vi "Dashboard Main (BEDPC-GB8-7's conflicted copy 2019-03-26).vi"() -> ()   [LabVIEW 2018]
uses:
  <vilib>/Utility/miscctls.llb/LVRowAndColumnTypeDef.ctl
  <vilib>/event_ctls.llb/eventvkey.ctl
  <vilib>/Rock Robotics/Network Tables/NT Read Boolean.vi
  <vilib>/Rock Robotics/Network Tables/NT Write Boolean.vi
  <vilib>/Rock Robotics/Network Tables/NT Read Numeric Array.vi
  <vilib>/Rock Robotics/WPI/Dashboard/WPI_DashboardLogging Global.vi
panel:
  in  "Camera Settings Right":T1={"Frame Rate"=30, "Compression"=30, "Size"=1, "DB Camera Config"=FALSE} {"Frame Rate" scale=1.0..30.0; "Compression" scale=100.0..-1.0; "Size" items=["640x480", "320x240", "160x120"]}
  in  "Camera Name Right":string(combo)="No Camera Selection"
  out "Camera Perf":string
  in  "Camera Settings":T1={"Frame Rate"=30, "Compression"=30, "Size"=1, "DB Camera Config"=FALSE} {"Frame Rate" scale=1.0..30.0; "Compression" scale=100.0..-1.0; "Size" items=["640x480", "320x240", "160x120"]}
  in  "TCP":refnum<k5>
  in  "Rec Mode":enum32{"Stop", "Record", "Playback"}(radio)
  out "Image Message":string="Timeout in Camera Communications"
  in  "Dashboard Tab":T2(tab)
  out "Limelight Target State":bool
  out "Hatch Open":bool
  out "Hatch Extend":bool
  out "Cargo Piston":bool
  in  "Zero Yaw":bool
  out "Yaw":dbl
  out "Cont Yaw":dbl
  out "LowerLimit":bool
  out "UpperLimit":bool
  out "HAB Retracting limit":bool
  out "HAB Extending limit":bool
  in  "Select Auto":string(combo)="Select Autonomous ..."
  out "NT Connection":bool
  out "Mode":T3(ring)=enum."Auto Disabled"
  out "Right Camera Perf":cluster{"Bandwidth (Mbps)":dbl, "FPS":dbl}
  out "Lift Auto Position":u16(ring) items=["Cargo 1", "Hatch 1", "Cargo 2", "Hatch 2", "Cargo 3", "Hatch 3"]
  out "Wheel Rates":T4
  out "Wheel Angles":T4
  out "Y-Velocity":dbl
  out "X-Velocity":dbl
  out "Wheel Positions":T4
  out "Tree":string(tree)
  in  "Test Slider":dbl(slide) scale=0.0..100.0 scale format="%#_3g"
  in  "On/Off":bool caption="Solenoid"
  in  "Test Name":u16(ring) items=["Select the test to run..."]
  in  "Test Tree":string(tree)
  in  "Motor":cluster{"Value":dbl, "Enable":bool} {"Value" scale=-1.0..1.0 scale format="%#_3g"}
  out "Progress":T5 {"Test Progress" scale=0.0..100.0}
  in  "Rev/Fwd":cluster{"Forward":bool, "Reverse":bool}
  in  "Test Ring":u16(ring) items=["Monochrome", "Color"]
  in  "CheckList":i32(listbox)
  out "Cmd Status":string
  in  "Execute Command":bool
  in  "Command Params":string[][](table)
  in  "Command Selection":i32(listbox)
  out "Camera Image":T6(plugin-control)
  in  "Camera Name":string(combo)="No Camera Selection"
  # "HW"
  # "HW"
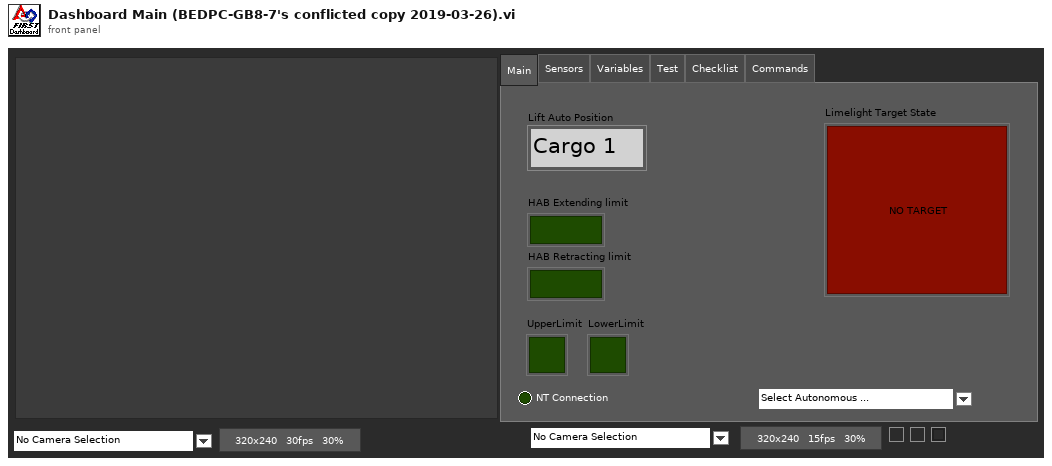
[diagram p1: front panel]
types:
  T1 = cluster{"Frame Rate":i32, "Compression":i32, "Size":u16, "DB Camera Config":bool}
  T2 = enum32{"Main", "Sensors", "Variables", "Test", "Checklist", "Commands"}
  T3 = enum8{"Tele-Op Disabled", "Tele-Op Enabled", "Auto Disabled", "Auto Enabled", "Test Disabled", "Test Enabled", "Disconnected", "No Code", "E-Stop"}
  T4 = cluster{"FrontLeft":dbl, "FrontRight":dbl, "BackLeft":dbl, "BackRight":dbl}
  T5 = cluster{"Test Progress":u8, "Test Progress Text":string}
  T6 = typedef "IMAQ Image.ctl" = refnum<image>
  T7 = cluster{"Save Path":path, "Interval (s)":dbl, "Keep":i32}
  T8 = enum32{"Drive", "Camera", "Basic", "Custom", "Test", "Commands", "Checklist", "Variables"}
  T9 = typedef "Image Type" = u32
  T10 = cluster{"IDs":cluster{"RPC field ID":u16, "Unique ID":u16}, "String":string}
  T11 = cluster{"Error Strings":string, "Disable Counts":cluster{u16, u16}, "Rail Faults":cluster{u16, u16, u16}, "Robot IP":string, "DB Mode":u8, "Event Info":cluster{"Name":string, "Type":u8, "Number":u16, "Replay":u8}}
  T12 = cluster{"Storage":cluster{"Disk Free":u64, "RAM Block":u32, "RAM free":u32}, "CPU Utilization":cluster{"CPU % ISR":sgl, "CPU % Time Crit":sgl, "CPU % Timed Str":sgl, "CPU % High":sgl, "CPU % Above":sgl, "CPU % Normal":sgl, "CPU % Low":sgl}, "CAN":cluster{"% Bus Utilization":sgl, "Bus Off Cnt":u32, "TX_FIFO Full Cnt":u32, "Receive Error Cnt":u8, "Transmit Error Cnt":u8}, "HID":cluster{"HID Outputs":u32, "Rumble Low":u16, "Rumble High":u16}[]}
  T13 = cluster{"Status bits":cluster{"Test Mode":bool, "Autonomous":bool, "Enabled":bool, "Code Start":bool, "Brownout":bool, "Reserved 2":bool, "Reserved 3":bool, "E-Stop":bool}, "Code Trace":cluster{"Disabled":bool, "TeleOp":bool, "Auto":bool, "Test":bool}, "Controller Type":enum16{"unknown", "cRIO", "roboRio"}, "Code?":enum16{"unknown", "noCode", "code"}, "Battery V":dbl}
  T14 = cluster{"Control Bits":cluster{"TestMode":bool, "Autonomous":bool, "Enabled":bool, "FMS Present":bool, bool, bool, bool, "E-Stop":bool}, "Team Station ":u8, "Countdown":sgl, "Joystick Values":cluster{"Axes":dbl[], "Buttons":bool[], "POVs":i16[]}[]}
  T15 = cluster{"Numeric":dbl, "Numeric":dbl, "Numeric":dbl, "Numeric":dbl}
  T16 = cluster{"Global Rectangle":i32[], "Contours":cluster{"Contour Type":u32, "ROI Type":u32, "Points":i32[]}[]}
  T17 = cluster{"Camera Name":string, string, "Saved DB Images Info":cluster{"Save Path":path, "Interval (s)":dbl, "Keep":i32}}
  T18 = cluster{"Camera Name Right":string, string, "Saved DB Images Info":cluster{"Save Path":path, "Interval (s)":dbl, "Keep":i32}}
  T19 = cluster{"Operation":enum16{"Update", "Clear"}, "Color Box":u32}[]
  T20 = typedef "eventvkey.ctl" = enum16{"ASCII", "Enter", "Return", "Shift", "Ctrl", "Alt", "Cmd", "Opt", "Caps", "NumLock", "Clear", "Break", "Up", "Down", "Left", "Right", "Insert", "Delete", "Home", "End", "PageUp", "PageDown", "Escape", "Help", "Pause", "ScrollLock", "F1", "F2", "F3", "F4", "F5", "F6", "F7", "F8", "F9", "F10", "F11", "F12", "F13", "F14", "F15", "F16", "F17", "F18", "F19", "F20", "F21", "F22", "F23", "F24", "Play", "VolumeUp", "VolumeDown", "Mute", "Two Byte Char"}
  T21 = cluster{"Operation":enum16{"Update", "Clear"}, "Color Box":u32}
  T22 = typedef "LVRowAndColumnTypeDef.ctl" = cluster{"Row":i32, "Column":i32}
  T23 = cluster{"Shift":bool, "Ctrl":bool, "Alt":bool, "Cmd":bool, "Opt":bool}
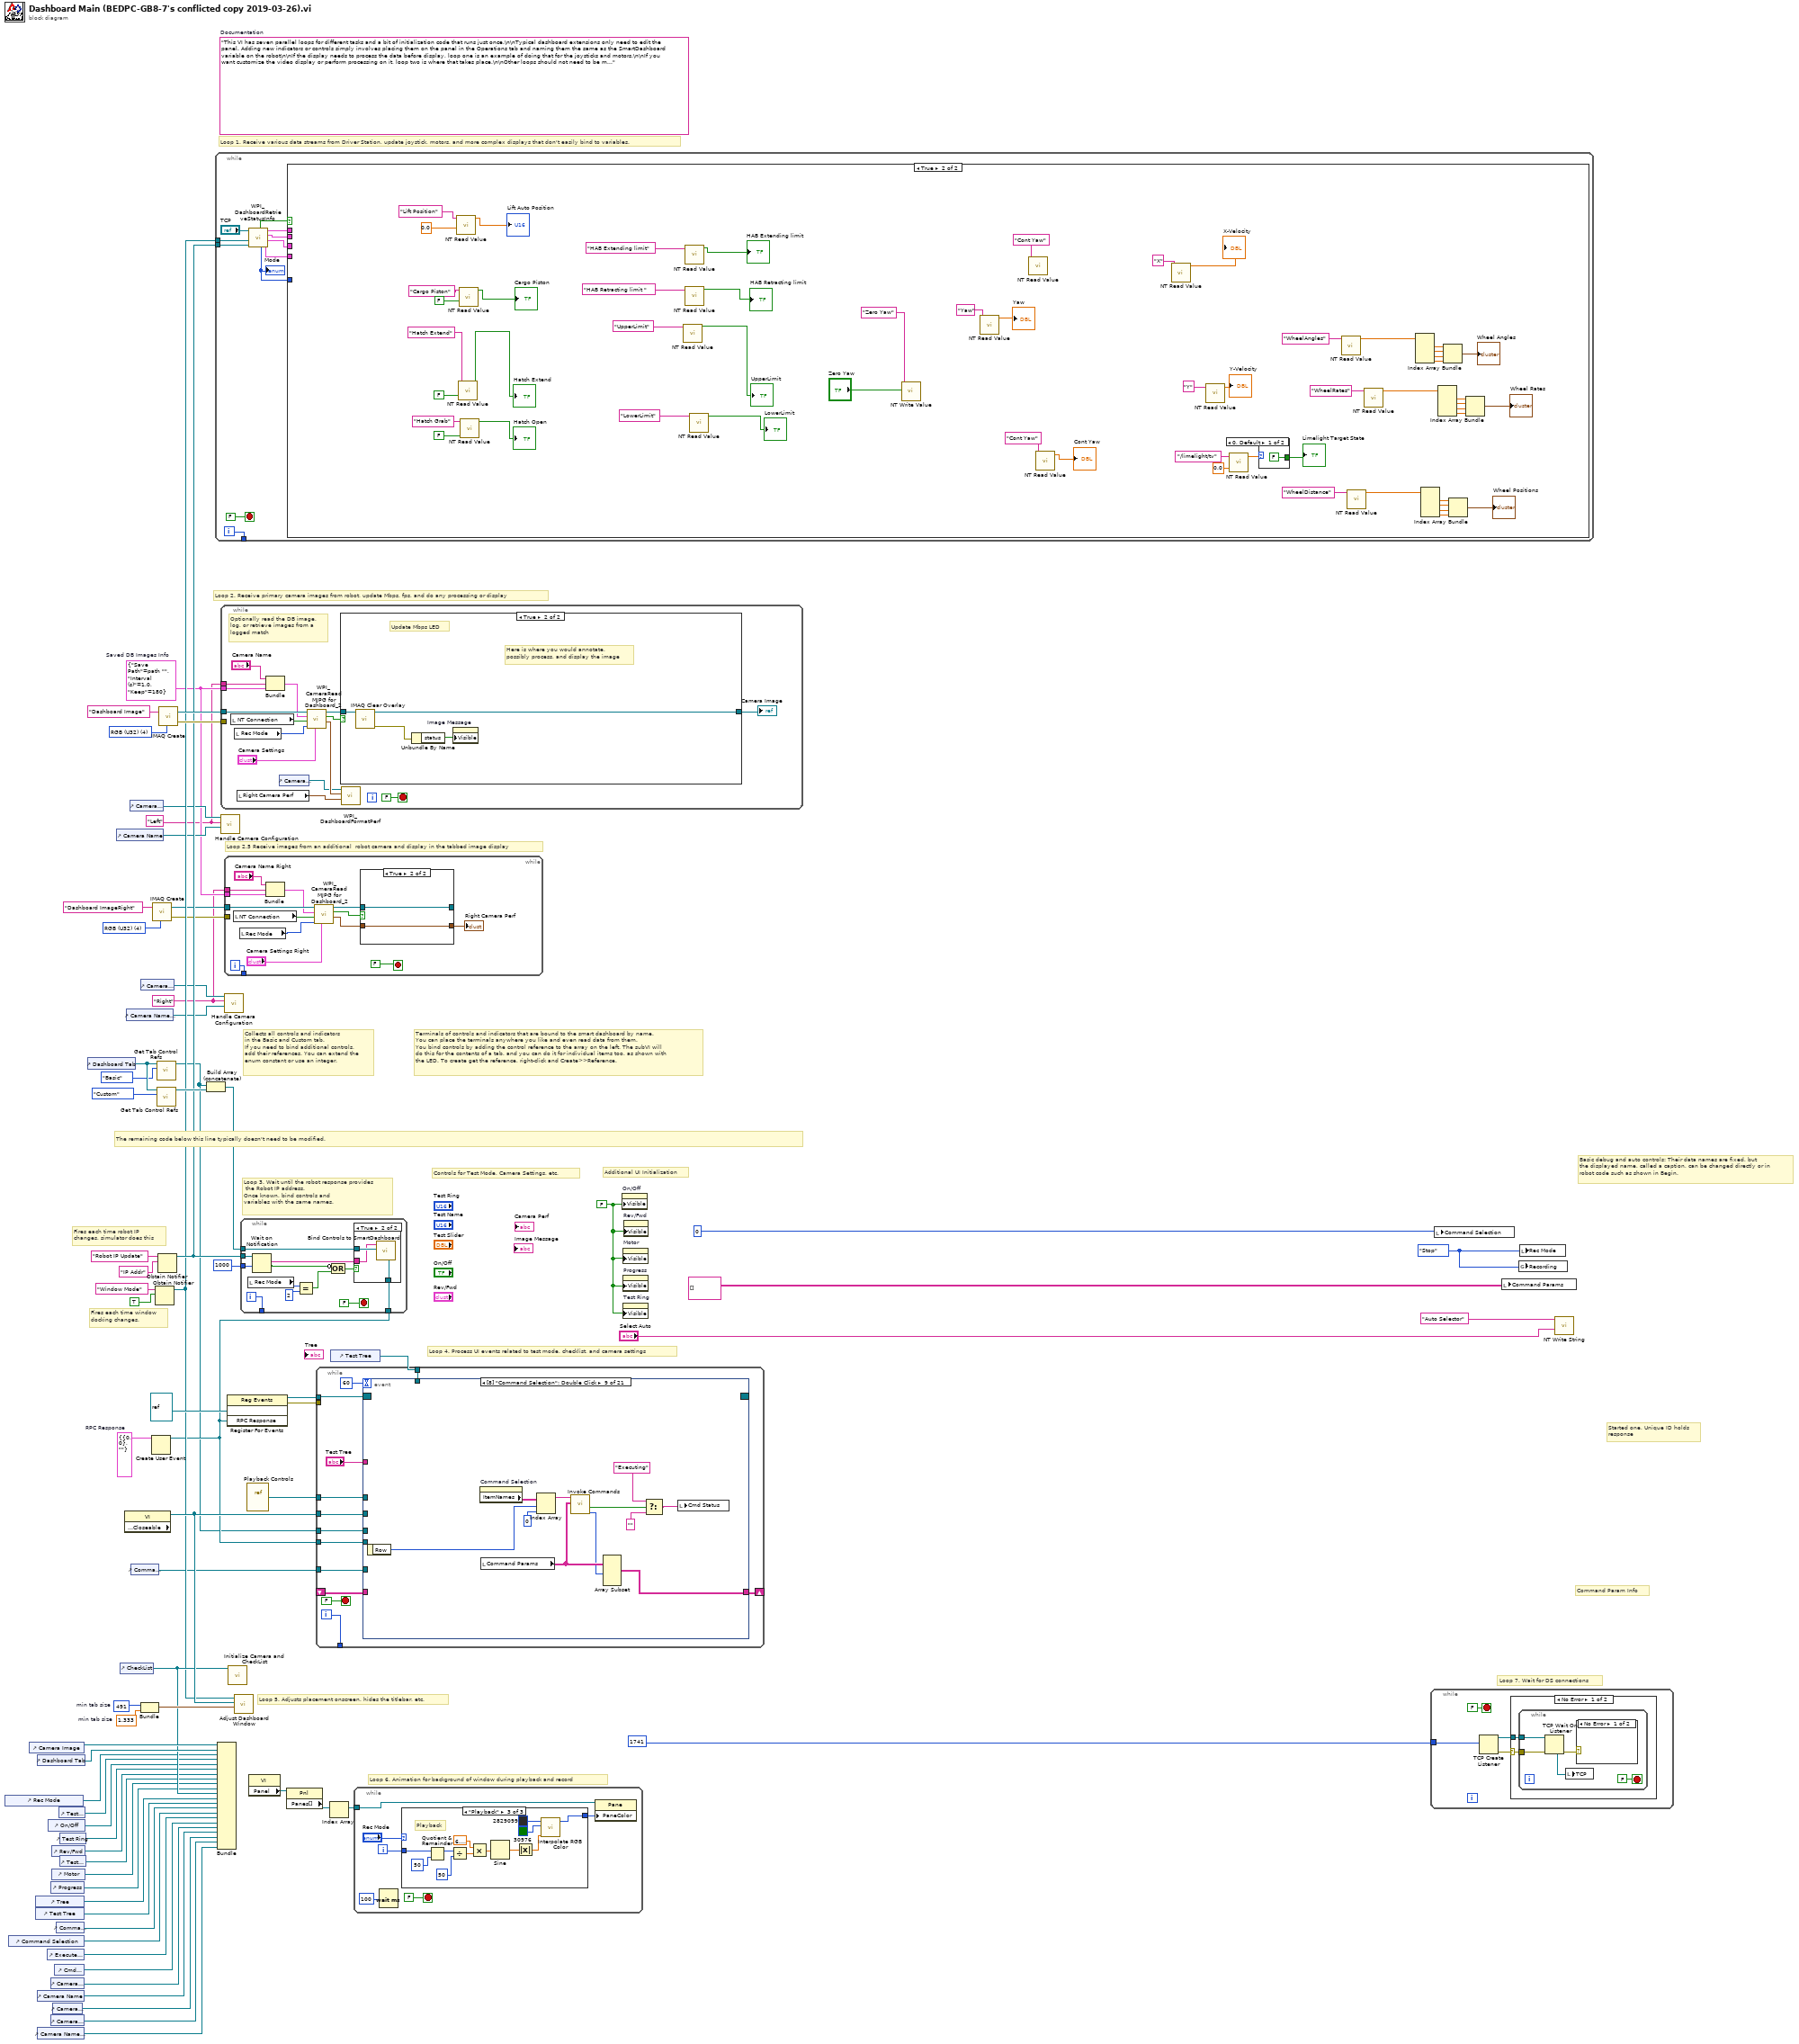
[diagram p0: block diagram]
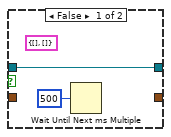
[diagram p2: hidden frame]
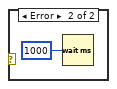
[diagram p3: hidden frame]
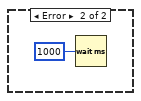
[diagram p4: hidden frame]
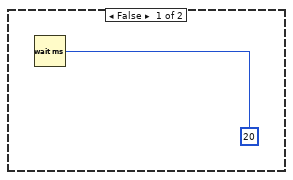
[diagram p5: hidden frame]
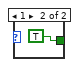
[diagram p6: hidden frame]
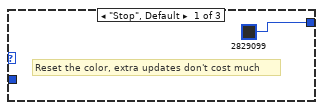
[diagram p7: hidden frame]
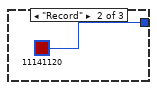
[diagram p8: hidden frame]
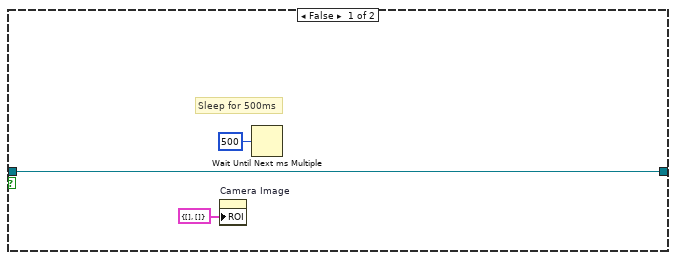
[diagram p10: hidden frame]
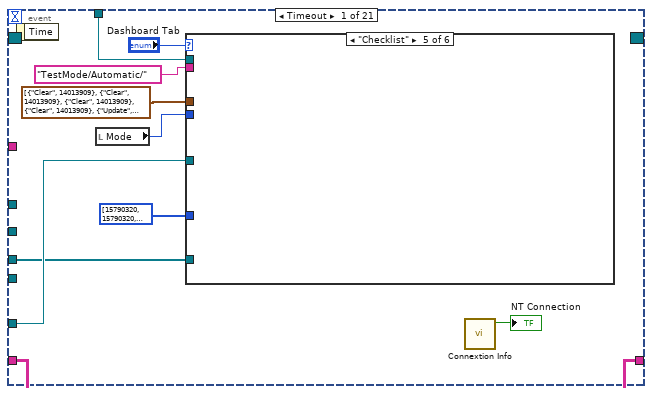
[diagram p11: hidden frame]
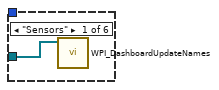
[diagram p12: hidden frame]
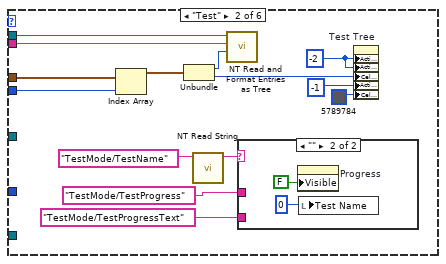
[diagram p13: hidden frame]
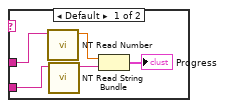
[diagram p14: hidden frame]
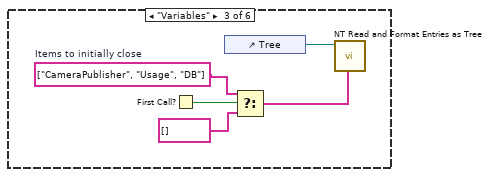
[diagram p15: hidden frame]
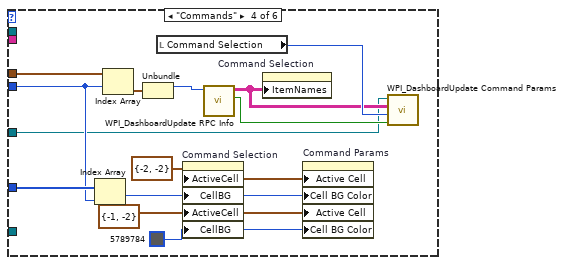
[diagram p16: hidden frame]
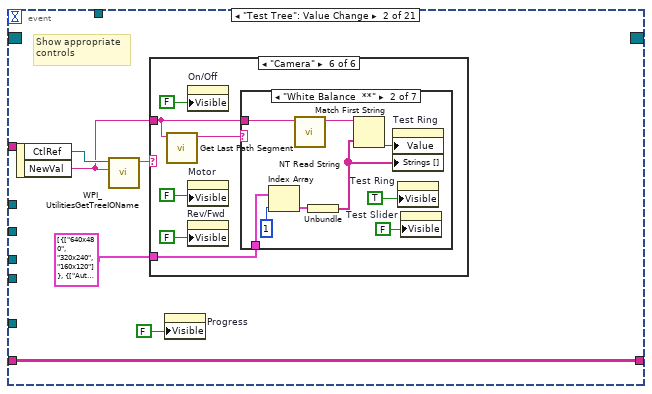
[diagram p18: hidden frame]
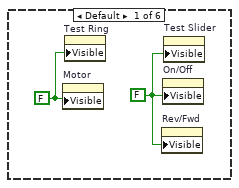
[diagram p19: hidden frame]
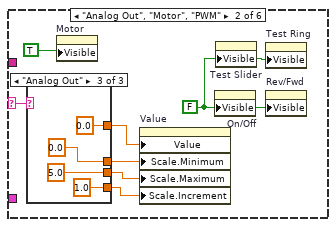
[diagram p20: hidden frame]
diagram:
  w3 = T7 {"Save Path"=path "", "Interval (s)"=1.0, "Keep"=180}  # Saved DB Images Info
  w2 = "Right"
  w1 = "Left"
  w12 = T9 4 items=["Grayscale (U8)", "Grayscale (I16)", "Grayscale (SGL)", "Complex (CSG)", "RGB (U32)", "HSL (U32)", "RGB (U64)"] ("Image Type")
  w28 = T10 {"IDs"={"RPC field ID"=0, "Unique ID"=0}, "String"=""}  # RPC Response
  w48 = 491  # min tab size
  w47 = 1.333  # min tab size
  w55 = enum32{"Stop", "Record", "Playback"}."Stop" ("Rec Mode")
  w34 = FALSE ("Visible")
  (unwired) "This VI has seven parallel loops for different tasks and a bit of initialization code that runs just once.\n\nTypical dashboard extensions only need to edit the panel. Adding new indicators or controls simply involves placing them on the panel in the Operations tab and naming them the same as the SmartDashboard variable on the robot\n\nIf the display needs to process the data before display, loop one is an example of doing that for the joysticks and motors.\n\nIf you want customize the video display or perform processing on it, loop two is where that takes place.\n\nOther loops should not need to be modified. They are pretty standard, and document the task they perform."  # Documentation
  w72 = T9 4 items=["Grayscale (U8)", "Grayscale (I16)", "Grayscale (SGL)", "Complex (CSG)", "RGB (U32)", "HSL (U32)", "RGB (U64)"] ("Image Type")
  # "Loop 2.5 Receive images from an additional  robot camera and display in the tabbed image display"
  # "Command Param Info"
  # "Started one, Unique ID holds\nresponse"
  # "Loop 7. Wait for DS connections"
  # "Basic debug and auto controls: Their data names are fixed, but\nthe displayed name, called a caption, can be changed directly or in\nrobot code such as shown in Begin."
  # "Controls for Test Mode, Camera Settings, etc."
  # "Additional UI Initialization"
  # "Loop 6. Animation for background of window during playback and record"
  # "Fires each time robot IP\nchanges, simulator does this"
  # "Fires each time window\ndocking changes."
  # "Collects all controls and indicators\nin the Basic and Custom tab.\nIf you need to bind additional controls,\nadd their references. You can extend the\nenum constant or use an integer."
  # "The remaining code below this line typically doesn't need to be modified."
  # "Loop 4. Process UI events related to test mode, checklist, and camera settings"
  # "Terminals of controls and indicators that are bound to the smart dashboard by name.\nYou can place the terminals anywhere you like and even read data from them.\nYou bind controls by adding the control reference to the array on the left. The subVI will\ndo this for the contents of a tab, and you can do it for individual items too, as shown with\nthe LED. To create get the reference, right-click and Create>>Reference."
  # "Loop 3. Wait until the robot response provides\n the Robot IP address.\nOnce known, bind controls and\nvariables with the same names."
  # "Loop 5. Adjusts placement onscreen, hides the titlebar, etc."
  # "Loop 1. Receive various data streams from Driver Station, update joystick, motors, and more complex displays that don't easily bind to variables."
  # "Loop 2. Receive primary camera images from robot, update Mbps, fps, and do any processing or display"
  n1 = control-ref of="Rec Mode"() -> (w40:refnum<vi>)
  n2 = control-ref of="Command Selection"() -> (w27:refnum<vi>)
  n3 = control-ref of="Camera Image"() -> (w50:refnum<vi>)
  n4 = control-ref of="Tree"() -> (w44:refnum<vi>)
  n5 = control-ref of="Test Tree"() -> (w43:refnum<vi>)
  n6 = control-ref of="Dashboard Tab"() -> (w49:refnum<vi>)
  n7 = control-ref of="Camera Name"() -> (w18:refnum<vi>)
  n8 = control-ref of="Camera Name Right"() -> (w6:refnum<vi>)
  n9 = control-ref of="Execute Command"() -> (w29:refnum<vi>)
  n10 = control-ref of="On/Off"() -> (w38:refnum<vi>)
  n11 = control-ref of="Progress"() -> (w35:refnum<vi>)
  n12 = control-ref of="Camera Settings"() -> (w19:refnum<vi>)
  n13 = control-ref of="Camera Settings Right"() -> (w7:refnum<vi>)
  n14 = control-ref of="Rev/Fwd"() -> (w36:refnum<vi>)
  n15 = control-ref of="Motor"() -> (w41:refnum<vi>)
  n16 = control-ref of="Camera Perf"() -> (w17:refnum<vi>)
  n17 = control-ref of="Cmd Status"() -> (w23:refnum<vi>)
  n18 = control-ref of="Command Params"() -> (w30:refnum<vi>)
  n19 = control-ref of="Test Slider"() -> (w39:refnum<vi>)
  n20 = control-ref of="Test Ring"() -> (w37:refnum<vi>)
  n21 = control-ref of="Test Name"() -> (w42:refnum<vi>)
  n22 = control-ref of="Dashboard Tab"() -> (w53:refnum<vi>)
  n23 = control-ref of="Camera Name"() -> (w20:refnum<vi>)
  n24 = control-ref of="CheckList"() -> (w45:refnum<vi>)
  n25 = property class="VI" props=["Front Panel.Closeable"]() -> (reference out=w54:refnum<vi>)  [unwired: 2 in, 2 out]
  n26 = control-ref of="Camera Name Right"() -> (w8:refnum<vi>)
  n27 = control-ref of="Camera Settings"() -> (w21:refnum<vi>)
  n28 = control-ref of="Command Params"() -> (w22:refnum<vi>)
  n29 = control-ref of="Camera Settings Right"() -> (w9:refnum<vi>)
  n30 = Bundle("min tab size"=w48, "min tab size"=w47) -> (w46:cluster{"min tab size":i32, "min tab size":dbl})  [unwired: 1 in]
  n31 = Create User Event(user event datatype=w28) -> (user event=w24:refnum<user-event>)  [unwired: 1 in, 1 out]
  n32 = call "IMAQ Create"("Image Name"="Dashboard ImageRight", "Image Type"=w12) -> ("New Image"=w11:T6, "error out"=w10:errorcluster)  [unwired: 2 in, 1 out]
  n33 = Obtain Notifier(name (unnamed)="Window Mode", notification data type=TRUE) -> (notifier out=w32:refnum<notifier>)  [unwired: 2 in, 2 out]
  n34 = call <vilib>:"Get Tab Control Refs.vi"("Page Index"=T8."Basic" ("Dashboard Tab"), "TabControl in"=w53) -> ("ControlsOnPage"=w16:refnum<vi>[])  [unwired: 9 in]
  n35 = call <vilib>:"Get Tab Control Refs.vi"("Page Index"=T8."Custom" ("Dashboard Tab"), "TabControl in"=w53) -> ("ControlsOnPage"=w52:refnum<vi>[])  [unwired: 9 in]
  n36 = Obtain Notifier(name (unnamed)="Robot IP Update", notification data type="IP Addr" ("name (unnamed)")) -> (notifier out=w33:refnum<notifier>)  [unwired: 2 in, 2 out]
  n37 = call "IMAQ Create"("Image Name"="Dashboard Image", "Image Type"=w72) -> ("New Image"=w70:T6, "error out"=w69:errorcluster)  [unwired: 2 in, 1 out]
  n38 = Build Array (concatenate)(w16, w52) -> (w51:refnum<vi>[])
  n39 = while {
    tunnel: [w82] -> _
    tunnel: w33 -> [w80]
    tunnel: w32 -> [w77]
    i -> [w82]
    stop <- FALSE stop-if-true
    n40 = call <vilib>:"WPI_DashboardRetrieveStatusInfo.vi"("Binding Refnum"=w80, "Window Mode Notifier"=w77, "TCP Cnx"="TCP") -> ("Power and Errors"=w74:T11, "Robot Metrics"=w73:T12, "Status Info"=w75:T13, "Control Info"=w76:T14, "Robot Mode"=w79:T3, "Process?"=w81:bool)  [unwired: 3 in]
    "Mode" <- w79
    n41 = case shown="True" w81 {
      tunnel: w79 -> [_ _]
      tunnel: w76 -> [_ _]
      tunnel: w75 -> [_ _]
      tunnel: w74 -> [_ _]
      tunnel: w73 -> [_ _]
      frame False {
        n42 = Wait (ms)(milliseconds to wait=u32 20) -> ()  [unwired: 1 out]
      }
      frame True {
        n43 = call-poly <vilib>:"NT Read Value.vi"("Default Value"=0.0, "Name"="Lift Position") -> ("Numeric"=→"Lift Auto Position":dbl)  [unwired: 8 in, 1 out]
        n44 = call-poly <vilib>:"NT Read Value.vi"("Default Value"=FALSE, "Name"="Hatch Extend") -> ("Boolean"=→"Hatch Extend":bool)  [unwired: 8 in, 1 out]
        n45 = call-poly <vilib>:"NT Read Value.vi"("Default Value"=FALSE, "Name"="Cargo Piston") -> ("Boolean"=→"Cargo Piston":bool)  [unwired: 8 in, 1 out]
        n46 = call-poly <vilib>:"NT Read Value.vi"("Default Value"=FALSE, "Name"="Hatch Grab") -> ("Boolean"=→"Hatch Open":bool)  [unwired: 8 in, 1 out]
        n47 = call-poly <vilib>:"NT Read Value.vi"("Name"="UpperLimit") -> ("Boolean"=→"UpperLimit":bool)  [unwired: 9 in, 1 out]
        n48 = call-poly <vilib>:"NT Read Value.vi"("Name"="HAB Extending limit") -> ("Boolean"=→"HAB Extending limit":bool)  [unwired: 9 in, 1 out]
        n49 = call-poly <vilib>:"NT Read Value.vi"("Name"="HAB Retracting limit ") -> ("Boolean"=→"HAB Retracting limit":bool)  [unwired: 9 in, 1 out]
        n50 = call-poly <vilib>:"NT Read Value.vi"("Name"="LowerLimit") -> ("Boolean"=→"LowerLimit":bool)  [unwired: 9 in, 1 out]
        n51 = call-poly <vilib>:"NT Write Value.vi"("Boolean"="Zero Yaw", "Name"="Zero Yaw") -> ()  [unwired: 9 in, 1 out]
        n52 = call-poly <vilib>:"NT Read Value.vi"("Name"="Yaw") -> ("Numeric"=→"Yaw":dbl)  [unwired: 9 in, 1 out]
        n53 = call-poly <vilib>:"NT Read Value.vi"("Name"="Cont Yaw") -> ()  [unwired: 9 in, 2 out]
        n54 = call-poly <vilib>:"NT Read Value.vi"("Name"="Cont Yaw") -> ("Numeric"=→"Cont Yaw":dbl)  [unwired: 9 in, 1 out]
        n55 = call-poly <vilib>:"NT Read Value.vi"("Name"="X") -> ("Numeric"=→"X-Velocity":dbl)  [unwired: 9 in, 1 out]
        n56 = call-poly <vilib>:"NT Read Value.vi"("Name"="Y") -> ("Numeric"=→"Y-Velocity":dbl)  [unwired: 9 in, 1 out]
        n57 = call-poly <vilib>:"NT Read Value.vi"("Default Value"=0.0, "Name"="/limelight/tv") -> ("Numeric"=w107:dbl)  [unwired: 8 in, 1 out]
        n58 = case shown="0, Default" w107 {
          tunnel: [FALSE TRUE] -> w106
          frame 0, Default {
          }
          frame 1 {
          }
        }
        "Limelight Target State" <- w106
        n59 = call-poly <vilib>:"NT Read Value.vi"("Name"="WheelAngles") -> ("Numeric Array"=w104:dbl[])  [unwired: 9 in, 1 out]
        n60 = call-poly <vilib>:"NT Read Value.vi"("Name"="WheelDistance") -> ("Numeric Array"=w89:dbl[])  [unwired: 9 in, 1 out]
        n61 = call-poly <vilib>:"NT Read Value.vi"("Name"="WheelRates") -> ("Numeric Array"=w94:dbl[])  [unwired: 9 in, 1 out]
        n62 = Index Array(array=w104) -> (element #1=w103:dbl, element #2=w102:dbl, element #3=w101:dbl, element #4=w100:dbl)  [unwired: 4 in]
        n63 = Index Array(array=w89) -> (element #1=w88:dbl, element #2=w87:dbl, element #3=w86:dbl, element #4=w85:dbl)  [unwired: 4 in]
        n64 = Index Array(array=w94) -> (element #1=w95:dbl, element #2=w96:dbl, element #3=w97:dbl, element #4=w98:dbl)  [unwired: 4 in]
        n65 = Bundle("Numeric"=w103, "Numeric"=w102, "Numeric"=w101, "Numeric"=w100) -> (→"Wheel Angles":T15)  [unwired: 1 in]
        n66 = Bundle("Numeric"=w88, "Numeric"=w87, "Numeric"=w86, "Numeric"=w85) -> (→"Wheel Positions":T15)  [unwired: 1 in]
        n67 = Bundle("Numeric"=w95, "Numeric"=w96, "Numeric"=w97, "Numeric"=w98) -> (→"Wheel Rates":T15)  [unwired: 1 in]
      }
    }
  }
  n68 = Bundle("Camera Image"=w50, "Dashboard Tab"=w49, "Rec Mode"=w40, "Test Slider"=w39, "On/Off"=w38, "Test Ring"=w37, "Rev/Fwd"=w36, "Test Name"=w42, "Motor"=w41, "Progress"=w35, "CheckList"=w45, "Tree"=w44, "Test Tree"=w43, "Command Params"=w30, "Command Selection"=w27, "Execute Command"=w29, "Cmd Status"=w23, "Camera Settings"=w19, "Camera Name"=w18, "Camera Perf"=w17, "Camera Settings Right"=w7, "Camera Name Right"=w6) -> ()  [unwired: 1 in, 1 out]
  n69 = call "Handle Camera Configuration.vi"("CameraNameRef"=w20, "Display Name"=w1, "ClusterRef"=w21) -> ()  [unwired: 9 in]
  n70 = while {
    tunnel: w70 -> [w156]
    tunnel: w69 -> [_]
    tunnel: w3 -> [w149]
    tunnel: w1 -> [w146]
    stop <- FALSE stop-if-true
    # "Optionally read the DB image,\nlog, or retrieve images from a\nlogged match"
    n71 = local read "NT Connection"() -> (w150:bool)
    n72 = local read "Rec Mode"() -> (w153:enum32{"Stop", "Record", "Playback"})
    n73 = local read "Right Camera Perf"() -> (w144:cluster{"Bandwidth (Mbps)":dbl, "FPS":dbl})
    n74 = Bundle("Camera Name"="Camera Name", w146, "Saved DB Images Info"=w149) -> (w148:T17)  [unwired: 1 in]
    n75 = control-ref of="Camera Perf"() -> (w143:refnum<vi>)
    n76 = call <vilib>:"WPI_CameraRead MJPG for Dashboard_2.vi"("Camera Settings"="Camera Settings", "Rec Mode"=w153, "NT Connection"=w150, "Capture Info"=w148, "Image in"=w156) -> ("perf info"=w145:cluster{"Bandwidth (Mbps)":dbl, "fps":dbl}, "Active"=w154:bool, "Image\\ out"=w155:T6)  [unwired: 4 in]
    n77 = case shown="True" w154 {
      tunnel: w155 -> [w159 w162]
      tunnel: [w159 w161] -> w151
      frame False {
        # "Sleep for 500ms"
        n78 = property on="Camera Image" class="ImageControl"("ROI"=T16 {"Global Rectangle"=[], "Contours"=[]}) -> ()  [unwired: 2 in, 2 out]
        n79 = Wait Until Next ms Multiple(millisecond multiple=u32 500) -> ()  [unwired: 1 out]
      }
      frame True {
        # "Here is where you would annotate,\npossibly process, and display the image"
        # "Update Mbps LED"
        n80 = call "IMAQ Clear Overlay"("Image"=w162) -> ("error out"=w163:errorcluster, "Image Out"=w161:T6)  [unwired: 2 in, 7 out]
        n81 = Unbundle By Name(w163) -> ("status"=w164:bool)
        n82 = property on="Image Message" class="Str"("Visible"=w164) -> ()  [unwired: 2 in, 2 out]
      }
    }
    "Camera Image" <- w151
    n83 = call <vilib>:"WPI_DashboardFormatPerf.vi"("Right Camera Perf"=w144, "Performance"=w145, "String in"=w143) -> ()  [unwired: 9 in]
  }
  n84 = call "Handle Camera Configuration.vi"("CameraNameRef"=w8, "Display Name"=w2, "ClusterRef"=w9) -> ()  [unwired: 9 in]
  n85 = while {
    tunnel: w11 -> [w178]
    tunnel: w10 -> [_]
    tunnel: [w173] -> _
    tunnel: w3 -> [w170]
    tunnel: w2 -> [w167]
    i -> [w173]
    stop <- FALSE stop-if-true
    n86 = local read "NT Connection"() -> (w171:bool)
    n87 = local read "Rec Mode"() -> (w177:enum32{"Stop", "Record", "Playback"})
    n88 = Bundle("Camera Name Right"="Camera Name Right", w167, "Saved DB Images Info"=w170) -> (w169:T18)  [unwired: 1 in]
    n89 = call <vilib>:"WPI_CameraRead MJPG for Dashboard_2.vi"("Camera Settings"="Camera Settings Right", "Rec Mode"=w177, "NT Connection"=w171, "Capture Info"=w169, "Image in"=w178) -> ("perf info"=w165:cluster{"Bandwidth (Mbps)":dbl, "fps":dbl}, "Active"=w172:bool, "Image\\ out"=w175:T6)  [unwired: 4 in]
    n90 = case shown="True" w172 {
      tunnel: w175 -> [w179 w182]
      tunnel: [w179 w182] -> _
      tunnel: [_ w181] -> w166
      tunnel: w165 -> [_ w181]
      frame False {
        (unwired) T16 {"Global Rectangle"=[], "Contours"=[]} ("ROI")
        n91 = Wait Until Next ms Multiple(millisecond multiple=u32 500) -> ()  [unwired: 1 out]
      }
      frame True {
      }
    }
    "Right Camera Perf" <- w166
  }
  n92 = register-events(refnum<vi> refnum, w24) -> (reference out=w59:refnum<event-registration>, error out=w58:errorcluster)  [unwired: 2 in]
  n93 = call "Initialize Camera and CheckList.vi"("ListBox in"=w45) -> ()  [unwired: 11 in]
  n94 = call "Adjust Dashboard Window.vi"("Size Constraints"=w46, "VI"=w54, "WIn Mode"=w32) -> ()  [unwired: 9 in]
  n95 = while {
    tunnel: w51 -> [w194]
    tunnel: w33 -> [w192]
    tunnel: [w190] -> _
    tunnel: u32 1000 ("milliseconds to wait") -> [w189]
    tunnel: w24 -> [w183]
    i -> [w190]
    stop <- FALSE stop-if-true
    n96 = local read "Rec Mode"() -> (w185:enum32{"Stop", "Record", "Playback"})
    n97 = Wait on Notification(notifier=w192, timeout in ms (-1)=w189) -> (notification=w191:string, timed out?=w187:bool)  [unwired: 2 in, 2 out]
    n98 = Equal?(x=w185, y=u16 2 ("Rec Mode")) -> (x = y?=w186:bool)
    n99 = Compound Arithmetic op=OR(invert w187, w186) -> (w188:bool)
    n100 = case shown="True" w188 {
      tunnel: w194 -> [_ w197]
      tunnel: w191 -> [_ w196]
      tunnel: w183 -> [_ w195]
      frame False {
      }
      frame True {
        n101 = call <vilib>:"Bind Controls to SmartDashboard.vi"("RPC ref"=w195, "Bound Control Refs"=w197, "Server IP Address"=w196) -> ()  [unwired: 9 in]
      }
    }
  }
  n102 = vi-ref "Playback Controls.vi"() -> (w60:refnum<vi>)
  n103 = property class="VI"() -> ("Panel"=w62:refnum<vi>)  [unwired: 2 in, 2 out]
  n104 = property class="Pnl"(reference=w62) -> ("Panes[]"=w63:refnum<vi>[])  [unwired: 1 in, 2 out]
  n105 = Index Array(array=w63) -> (element=w61:refnum<vi>)  [unwired: 1 in]
  n106 = control-ref of="Test Tree"() -> (w64:refnum<vi>)
  n107 = while {
    tunnel: [w207] -> _
    tunnel: w64 -> [w206]
    tunnel: w60 -> [w205]
    tunnel: w59 -> [w204]
    tunnel: w58 -> [_]
    tunnel: w54 -> [w203]
    tunnel: w24 -> [w202]
    tunnel: w22 -> [w201]
    shift-right: [w200] -> _
    shift-left: _ -> [w199]
    tunnel: w16 -> [w198]
    i -> [w207]
    stop <- FALSE stop-if-true
    n108 = event shown="[8] \"Command Selection\": Double Click" {
      selector: w204 -> [_ _ _ _ _ _ _ _ _ _ _ _ _ _ _ _ _ _ _ _ _]
      dyn-events: [_ _ _ _ _ _ _ _ _ _ _ _ _ _ _ _ w465 _ _ _ _] -> _
      timeout: u32 60 ("milliseconds to wait") -> [_ _ _ _ _ _ _ _ _ _ _ _ _ _ _ _ _ _ _ _ _]
      tunnel: w206 -> [w219 _ _ _ _ _ _ _ _ _ _ _ _ _ _ _ _ _ _ _ _]
      tunnel: "Test Tree" -> [_ _ _ _ _ _ _ _ _ _ _ w434 w442 w444 w448 w456 _ _ _ _ _]
      tunnel: w205 -> [_ _ _ _ _ _ _ _ _ _ _ _ _ _ _ _ w467 _ w483 _ _]
      tunnel: w203 -> [_ _ _ _ _ _ _ _ _ _ _ _ _ _ _ _ w463 _ _ _ _]
      tunnel: w202 -> [_ _ _ _ _ _ _ _ _ _ _ _ _ _ _ _ w461 _ _ _ _]
      tunnel: w201 -> [w214 _ _ _ _ _ w385 _ _ _ _ _ _ _ _ _ _ _ _ _ _]
      tunnel: [w213 w262 w364 w369 w378 w382 w383 w392 w402 w409 w421 w433 w440 w443 w447 w455 w460 w478 w480 w484 w497] -> w200
      tunnel: w199 -> [w213 w262 w364 w369 w378 w382 w383 _ _ w409 w421 w433 w440 w443 w447 w455 w460 w478 w480 w484 w497]
      tunnel: w198 -> [w211 _ _ _ _ _ _ _ _ _ _ _ _ _ _ _ _ _ _ _ _]
      event Timeout {
        n109 = event-data() -> ()  [unwired: 1 in, 1 out]
        n110 = local read "Mode"() -> (w216:T3)
        n111 = case shown="\"Checklist\"" "Dashboard Tab" {
          tunnel: w219 -> [_ w235 _ _ _ _]
          tunnel: "TestMode/Automatic/" ("Name Pattern") -> [_ w234 _ _ _ _]
          tunnel: T19 [{"Operation"=enum."Clear", "Color Box"=14013909}, {"Operation"=enum."Clear", "Color Box"=14013909}, {"Operation"=enum."Clear", "Color Box"=14013909}, {"Operation"=enum."Clear", "Color Box"=14013909}, {"Operation"=enum."Update", "Color Box"=14013909}, {"Operation"=enum."Update", "Color Box"=16777215}, {"Operation"=enum."Clear", "Color Box"=14013909}, {"Operation"=enum."Clear", "Color Box"=14013909}, {"Operation"=enum."Clear", "Color Box"=14013909}] -> [_ w227 _ w255 _ _]
          tunnel: w216 -> [_ w226 _ w254 _ _]
          tunnel: u32[] [15790320, 15790320, 15790320, 15790320, 16777215, 16777215, 15790320, 15790320, 15790320] -> [_ _ _ w260 _ _]
          tunnel: w214 -> [_ _ _ w248 _ _]
          tunnel: w211 -> [w221 _ _ _ _ _]
          frame "Sensors" {
            n112 = call <vilib>:"WPI_DashboardUpdateNames.vi"("Controls on Tab"=w221) -> ()  [unwired: 11 in]
          }
          frame "Test" {
            w233 = -2 ("Active Item:Row Number")
            n113 = Index Array(array=w227, index=w226) -> (element=w228:T21)
            n114 = Unbundle(w228) -> ("Operation"=w229:enum16{"Update", "Clear"}, "Color Box"=w230:u32)
            n115 = call <vilib>:"NT Read String.vi"("Name"="TestMode/TestName") -> ("String"=w224:string)  [unwired: 9 in, 1 out]
            n116 = call <vilib>:"NT Read and Format Entries as Tree.vi"("Operation"=w229, "Name Pattern"=w234, "Tree Refnum"=w235) -> ()  [unwired: 7 in, 2 out]
            n117 = case shown="\"\"" w224 {
              tunnel: "TestMode/TestProgress" ("Name") -> [w237 _]
              tunnel: "TestMode/TestProgressText" ("Name") -> [w236 _]
              frame Default {
                n118 = call <vilib>:"NT Read Number.vi"("Name"=w237) -> ("Numeric"=w238:dbl)  [unwired: 9 in, 1 out]
                n119 = call <vilib>:"NT Read String.vi"("Name"=w236) -> ("String"=w239:string)  [unwired: 9 in, 1 out]
                n120 = Bundle("Numeric"=w238, "String"=w239) -> (→"Progress":cluster{"Numeric":dbl, "String":string})  [unwired: 1 in]
              }
              frame "" {
                n121 = property on="Progress" class="Clust (strict)"("Visible"=FALSE) -> ()  [unwired: 2 in, 2 out]
                n122 = local write "Test Name"(u16 0) -> ()
              }
            }
            n123 = property on="Test Tree" class="Tree (strict)"("Active Item Row Number"=w233, "ActiveColNum"=w233, "CellBG"=w230, "Active Item Row Number"=-1 ("Active Item:Row Number"), "CellBG"=u32 5789784 ("Color Box")) -> ()  [unwired: 2 in, 2 out]
          }
          frame "Variables" {
            w245 = string[] ["CameraPublisher", "Usage", "DB"]  # Items to initially close
            n124 = First Call?() -> (First Call?: T/F=w246:bool)
            n125 = control-ref of="Tree"() -> (w247:refnum<vi>)
            n126 = Select(t=w245, s=w246, f=string[] []) -> (s? t:f=w243:string[])
            n127 = call <vilib>:"NT Read and Format Entries as Tree.vi"("Tags to  Close"=w243, "Tree Refnum"=w247) -> ()  [unwired: 8 in, 2 out]
          }
          frame "Commands" {
            w256 = u32 5789784 ("Color Box")
            w257 = T22 {"Row"=-1, "Column"=-2} ("Active Cell:Active Cell")
            w259 = T22 {"Row"=-2, "Column"=-2} ("Active Cell:Active Cell")
            n128 = Index Array(array=w260, index=w254) -> (element=w258:u32)
            n129 = Index Array(array=w255, index=w254) -> (element=w253:T21)
            n130 = Unbundle(w253) -> ("Operation"=w252:enum16{"Update", "Clear"})  [unwired: 1 out]
            n131 = local read "Command Selection"() -> (w251:i32)
            n132 = property on="Command Selection" class="MCListbox (strict)"("ActiveCell"=w259, "CellBG"=w258, "ActiveCell"=w257, "CellBG"=w256) -> ()  [unwired: 2 in, 2 out]
            n133 = call <vilib>:"WPI_DashboardUpdate RPC Info.vi"("Operation"=w252) -> ("update"=w250:bool, "commands"=w249:string[][])  [unwired: 9 in]
            n134 = property on="Command Selection" class="MCListbox (strict)"("ItemNames"=w249) -> ()  [unwired: 2 in, 2 out]
            n135 = property on="Command Params" class="Tbl (strict)"("Active Cell"=w259, "Cell BG Color"=w258, "Active Cell"=w257, "Cell BG Color"=w256) -> ()  [unwired: 2 in, 2 out]
            n136 = call <vilib>:"WPI_DashboardUpdate Command Params.vi"("Update"=w250, "NewVal"=w251, "Commands"=w249, "Param Tbl"=w248) -> ()  [unwired: 7 in, 1 out]
          }
          frame "Checklist" {
          }
          frame "Main" {
          }
        }
        n137 = call <vilib>:"Connextion Info.vi"() -> ("Connected"=→"NT Connection":bool)  [unwired: 10 in, 1 out]
      }
      event "Test Tree": Value Change {
        # "Show appropriate\ncontrols"
        n138 = event-data() -> ("CtlRef"=w265:refnum<vi>, "NewVal"=w263:string)  [unwired: 1 in]
        n139 = call <vilib>:"WPI_UtilitiesGetTreeIOName.vi"("NewVal"=w263, "TreeControl in"=w265) -> ("I/O Name"=w266:string)  [unwired: 9 in]
        n140 = case shown="\"Camera\"" w266 {
          selector: w266 -> [_ w273 _ w295 w304 _]
          tunnel: w263 -> [_ _ w292 w294 _ w311]
          tunnel: cluster{string[]}[] [{["640x480", "320x240", "160x120"]}, {["Auto", "Fixed indoor", "Fixed outdoor 1", "Fixed outdoor 2", "Fixed fluorescent 1", "Fixed fluorescent 2", "Hold current"]}, {["Auto", "Flicker-free 50 Hz", "Flicker-free 60 Hz", "Hold current"]}, {["None", "Prioritize frame rate", "Prioritize image quality"]}, {["Monochrome", "Color"]}] -> [_ _ _ _ _ w310]
          frame Default {
            w268 = FALSE ("Visible")
            w267 = FALSE ("Visible")
            n141 = property on="Motor" class="Clust (strict)"("Visible"=w267) -> ()  [unwired: 2 in, 2 out]
            n142 = property on="Test Ring" class="Ring (strict)"("Visible"=w267) -> ()  [unwired: 2 in, 2 out]
            n143 = property on="Rev/Fwd" class="Clust (strict)"("Visible"=w268) -> ()  [unwired: 2 in, 2 out]
            n144 = property on="On/Off" class="Bool (strict)"("Visible"=w268) -> ()  [unwired: 2 in, 2 out]
            n145 = property on="Test Slider" class="Slide (strict)"("Visible"=w268) -> ()  [unwired: 2 in, 2 out]
          }
          frame "Analog Out", "Motor", "PWM" {
            w274 = FALSE ("Visible")
            n146 = case shown="\"Analog Out\"" w273 {
              tunnel: [1.0 ("Value") -1.0 ("Value") 0.0 ("Value")] -> w272
              tunnel: [255.0 ("Value") 1.0 ("Value") 5.0 ("Value")] -> w271
              tunnel: [128.0 ("Value") 0.0 ("Value") 0.0 ("Value")] -> w270
              tunnel: [64.0 ("Value") 0.5 ("Value") 1.0 ("Value")] -> w269
              frame "PWM" {
              }
              frame "Motor", Default {
              }
              frame "Analog Out" {
              }
            }
            n147 = property on="Motor" class="Clust (strict)"("Visible"=TRUE) -> ()  [unwired: 2 in, 2 out]
            n148 = property on="Value" class="Slide (strict)"("Value"=w270, "Scale.Minimum"=w272, "Scale.Maximum"=w271, "Scale.Increment"=w269) -> ()  [unwired: 2 in, 2 out]
            n149 = property on="On/Off" class="Bool (strict)"("Visible"=w274) -> ()  [unwired: 2 in, 2 out]
            n150 = property on="Test Slider" class="Slide (strict)"("Visible"=w274) -> ()  [unwired: 2 in, 2 out]
            n151 = property on="Test Ring" class="Ring (strict)"("Visible"=w274) -> ()  [unwired: 2 in, 2 out]
            n152 = property on="Rev/Fwd" class="Clust (strict)"("Visible"=w274) -> ()  [unwired: 2 in, 2 out]
          }
          frame "Servo" {
            w290 = FALSE ("Visible")
            n153 = call <vilib>:"NT Read Number.vi"("Name"=w292) -> ("Numeric"=w291:dbl)  [unwired: 9 in, 1 out]
            n154 = property on="Test Slider" class="Slide (strict)"("Visible"=TRUE, "Scale.Maximum"=170.0 ("Scale.Range:Maximum")) -> ()  [unwired: 2 in, 2 out]
            n155 = local write "Test Slider"(w291) -> ()
            n156 = property on="Motor" class="Clust (strict)"("Visible"=w290) -> ()  [unwired: 2 in, 2 out]
            n157 = property on="Rev/Fwd" class="Clust (strict)"("Visible"=w290) -> ()  [unwired: 2 in, 2 out]
            n158 = property on="On/Off" class="Bool (strict)"("Visible"=w290) -> ()  [unwired: 2 in, 2 out]
            n159 = property on="Test Ring" class="Ring (strict)"("Visible"=w290) -> ()  [unwired: 2 in, 2 out]
          }
          frame "Relay", "Solenoid" {
            w293 = FALSE ("Visible")
            n160 = property on="Motor" class="Clust (strict)"("Visible"=w293) -> ()  [unwired: 2 in, 2 out]
            n161 = property on="Test Slider" class="Slide (strict)"("Visible"=w293) -> ()  [unwired: 2 in, 2 out]
            n162 = Search and Replace String(input string=w294, search string="/Value  **", replace string="/Direction") -> (result string=w300:string)  [unwired: 5 in, 3 out]
            n163 = property on="Test Ring" class="Ring (strict)"("Visible"=w293) -> ()  [unwired: 2 in, 2 out]
            n164 = call <vilib>:"NT Read String.vi"("Name"=w300) -> ("String"=w298:string)  [unwired: 9 in, 1 out]
            n165 = Equal?(x="Both directions", y=w298) -> (x = y?=w296:bool)
            n166 = Not(x=w296) -> (.not. x?=w297:bool)
            n167 = property on="Rev/Fwd" class="Clust (strict)"("Visible"=w296) -> ()  [unwired: 2 in, 2 out]
            n168 = property on="On/Off" class="Bool (strict)"("Visible"=w297, "Caption.Text"=w295) -> ()  [unwired: 2 in, 2 out]
          }
          frame "Compressor", "Digital Out" {
            w303 = FALSE ("Visible")
            # "Get direction and finish"
            n169 = property on="Motor" class="Clust (strict)"("Visible"=w303) -> ()  [unwired: 2 in, 2 out]
            n170 = property on="Test Slider" class="Slide (strict)"("Visible"=w303) -> ()  [unwired: 2 in, 2 out]
            n171 = property on="Test Ring" class="Ring (strict)"("Visible"=w303) -> ()  [unwired: 2 in, 2 out]
            n172 = property on="On/Off" class="Bool (strict)"("Visible"=TRUE, "Caption.Text"=w304) -> ()  [unwired: 2 in, 2 out]
            n173 = property on="Rev/Fwd" class="Clust (strict)"("Visible"=FALSE) -> ()  [unwired: 2 in, 2 out]
          }
          frame "Camera" {
            n174 = call <vilib>:"Get Last Path Segment.vi"("String in"=w311) -> ("String out"=w312:string)  [unwired: 10 in]
            n175 = property on="On/Off" class="Bool (strict)"("Visible"=FALSE) -> ()  [unwired: 2 in, 2 out]
            n176 = property on="Motor" class="Clust (strict)"("Visible"=FALSE) -> ()  [unwired: 2 in, 2 out]
            n177 = property on="Rev/Fwd" class="Clust (strict)"("Visible"=FALSE) -> ()  [unwired: 2 in, 2 out]
            n178 = case shown="\"White Balance  **\"" w312 {
              tunnel: w311 -> [w318 w327 w336 w345 w354 _ w360]
              tunnel: w310 -> [w316 w324 w333 w342 w351 _ _]
              frame "Size  **" {
                n179 = Index Array(array=w316) -> (element=w315:cluster{string[]})  [unwired: 1 in]
                n180 = call <vilib>:"NT Read String.vi"("Name"=w318) -> ("String"=w317:string)  [unwired: 9 in, 1 out]
                n181 = Unbundle(w315) -> (w313:string[])
                n182 = Match First String(2:w313, 3:w317) -> (0:w314:i32)  [unwired: 1 out]
                n183 = property on="Test Ring" class="Ring (strict)"("Value"=w314, "Strings []"=w313) -> ()  [unwired: 2 in, 2 out]
                n184 = property on="Test Ring" class="Ring (strict)"("Visible"=TRUE) -> ()  [unwired: 2 in, 2 out]
                n185 = property on="Test Slider" class="Slide (strict)"("Visible"=FALSE) -> ()  [unwired: 2 in, 2 out]
              }
              frame "White Balance  **" {
                n186 = Index Array(array=w324, index=1) -> (element=w325:cluster{string[]})
                n187 = call <vilib>:"NT Read String.vi"("Name"=w327) -> ("String"=w326:string)  [unwired: 9 in, 1 out]
                n188 = Unbundle(w325) -> (w322:string[])
                n189 = Match First String(2:w322, 3:w326) -> (0:w321:i32)  [unwired: 1 out]
                n190 = property on="Test Ring" class="Ring (strict)"("Value"=w321, "Strings []"=w322) -> ()  [unwired: 2 in, 2 out]
                n191 = property on="Test Ring" class="Ring (strict)"("Visible"=TRUE) -> ()  [unwired: 2 in, 2 out]
                n192 = property on="Test Slider" class="Slide (strict)"("Visible"=FALSE) -> ()  [unwired: 2 in, 2 out]
              }
              frame "Exposure  **" {
                n193 = Index Array(array=w333, index=2) -> (element=w334:cluster{string[]})
                n194 = call <vilib>:"NT Read String.vi"("Name"=w336) -> ("String"=w335:string)  [unwired: 9 in, 1 out]
                n195 = Unbundle(w334) -> (w330:string[])
                n196 = Match First String(2:w330, 3:w335) -> (0:w331:i32)  [unwired: 1 out]
                n197 = property on="Test Ring" class="Ring (strict)"("Value"=w331, "Strings []"=w330) -> ()  [unwired: 2 in, 2 out]
                n198 = property on="Test Ring" class="Ring (strict)"("Visible"=TRUE) -> ()  [unwired: 2 in, 2 out]
                n199 = property on="Test Slider" class="Slide (strict)"("Visible"=FALSE) -> ()  [unwired: 2 in, 2 out]
              }
              frame "Exposure Priority  **" {
                n200 = Index Array(array=w342, index=3) -> (element=w343:cluster{string[]})
                n201 = call <vilib>:"NT Read String.vi"("Name"=w345) -> ("String"=w344:string)  [unwired: 9 in, 1 out]
                n202 = Unbundle(w343) -> (w339:string[])
                n203 = Match First String(2:w339, 3:w344) -> (0:w340:i32)  [unwired: 1 out]
                n204 = property on="Test Ring" class="Ring (strict)"("Value"=w340, "Strings []"=w339) -> ()  [unwired: 2 in, 2 out]
                n205 = property on="Test Ring" class="Ring (strict)"("Visible"=TRUE) -> ()  [unwired: 2 in, 2 out]
                n206 = property on="Test Slider" class="Slide (strict)"("Visible"=FALSE) -> ()  [unwired: 2 in, 2 out]
              }
              frame "Color Enable  **" {
                n207 = Index Array(array=w351, index=4) -> (element=w352:cluster{string[]})
                n208 = call <vilib>:"NT Read String.vi"("Name"=w354) -> ("String"=w353:string)  [unwired: 9 in, 1 out]
                n209 = Unbundle(w352) -> (w348:string[])
                n210 = Match First String(2:w348, 3:w353) -> (0:w349:i32)  [unwired: 1 out]
                n211 = property on="Test Ring" class="Ring (strict)"("Value"=w349, "Strings []"=w348) -> ()  [unwired: 2 in, 2 out]
                n212 = property on="Test Ring" class="Ring (strict)"("Visible"=TRUE) -> ()  [unwired: 2 in, 2 out]
                n213 = property on="Test Slider" class="Slide (strict)"("Visible"=FALSE) -> ()  [unwired: 2 in, 2 out]
              }
              frame Default {
                n214 = property on="Test Ring" class="Ring (strict)"("Visible"=FALSE) -> ()  [unwired: 2 in, 2 out]
                n215 = property on="Test Slider" class="Slide (strict)"("Visible"=FALSE) -> ()  [unwired: 2 in, 2 out]
              }
              frame "Brightness  **", "Color Level  **", "Compression  **", "FPS  **", "Sharpness  **" {
                n216 = call <vilib>:"NT Read Number.vi"("Name"=w360) -> ("Numeric"=w359:dbl)  [unwired: 9 in, 1 out]
                n217 = local write "Test Slider"(w359) -> ()
                n218 = property on="Test Slider" class="Slide (strict)"("Visible"=TRUE, "Scale.Maximum"=100.0 ("Scale.Range:Maximum")) -> ()  [unwired: 2 in, 2 out]
                n219 = property on="Test Ring" class="Ring (strict)"("Visible"=FALSE) -> ()  [unwired: 2 in, 2 out]
              }
            }
          }
        }
        n220 = property on="Progress" class="Clust (strict)"("Visible"=FALSE) -> ()  [unwired: 2 in, 2 out]
      }
      event "Test Name": Mouse Enter {
        # "Populate the ring with the list of tests"
        n221 = event-data() -> ()  [unwired: 1 in, 1 out]
        n222 = call <vilib>:"NT Read String Array.vi"("Name"="TestMode/TestList") -> ("String Array"=w368:string[])  [unwired: 9 in, 1 out]
        n223 = Build Array (concatenate)("Select the test to run...", w368) -> (w367:string[])
        n224 = property on="Test Name" class="Ring (strict)"("Strings []"=w367) -> ()  [unwired: 2 in, 2 out]
      }
      event "Test Name": Value Change {
        w370 = FALSE ("Visible")
        # "Tell the robot the test name to run"
        n225 = event-data() -> ("NewVal"=w374:u16)  [unwired: 1 in]
        n226 = property on="Test Name" class="Ring (strict)"() -> ("Strings []"=w375:string[])  [unwired: 2 in, 2 out]
        n227 = local write "Progress"(T5 {"Test Progress"=0, "Test Progress Text"=""} ("Progress")) -> ()
        n228 = Index Array(array=w375, index=w374) -> (element=w373:string)
        n229 = call <vilib>:"NT Write String.vi"("String"=w373, "Name"="TestMode/TestName") -> ()  [unwired: 9 in, 1 out]
        n230 = property on="Progress" class="Clust (strict)"("Visible"=TRUE) -> ()  [unwired: 2 in, 2 out]
        n231 = property on="Motor" class="Clust (strict)"("Visible"=w370) -> ()  [unwired: 2 in, 2 out]
        n232 = property on="Test Slider" class="Slide (strict)"("Visible"=w370) -> ()  [unwired: 2 in, 2 out]
        n233 = property on="On/Off" class="Bool (strict)"("Visible"=w370) -> ()  [unwired: 2 in, 2 out]
        n234 = property on="Rev/Fwd" class="Clust (strict)"("Visible"=w370) -> ()  [unwired: 2 in, 2 out]
        n235 = property on="Test Ring" class="Ring (strict)"("Visible"=w370) -> ()  [unwired: 2 in, 2 out]
      }
      event "Select Auto": Mouse Enter {
        # "Populate the combo box with the list of autonomous options"
        n236 = event-data() -> ()  [unwired: 1 in, 1 out]
        n237 = call <vilib>:"NT Read String Array.vi"("Name"="Auto List") -> ("String Array"=w377:string[])  [unwired: 9 in, 1 out]
        n238 = property on="Select Auto" class="CmbBox"("Strings[]"=w377) -> ()  [unwired: 2 in, 2 out]
      }
      event "Select Auto": Value Change {
        # "User modified the Auto Selection. Write to NT variable so robot knows."
        n239 = event-data() -> ("NewVal"=w380:string)  [unwired: 1 in]
        n240 = call <vilib>:"NT Write String.vi"("String"=w380, "Name"="Auto Selector") -> ()  [unwired: 9 in, 1 out]
      }
      event "Command Selection": Value Change {
        # "Get the params and show in table"
        n241 = event-data() -> ("NewVal"=w386:i32)  [unwired: 1 in]
        n242 = property on="Command Selection" class="MCListbox (strict)"() -> ("ItemNames"=w384:string[][])  [unwired: 2 in, 2 out]
        n243 = call <vilib>:"WPI_DashboardUpdate Command Params.vi"("NewVal"=w386, "Commands"=w384, "Param Tbl"=w385) -> ()  [unwired: 8 in, 1 out]
      }
      event "Execute Command": Value Change {
        # "Started one, Unique ID holds\nresponse"
        n244 = event-data() -> ()  [unwired: 1 in, 1 out]
        n245 = property on="Command Selection" class="MCListbox (strict)"() -> ("ItemNames"=w397:string[][])  [unwired: 2 in, 2 out]
        n246 = Index Array(array=w397, index (row)="Command Selection", index (col)=0) -> (element=w395:string)
        n247 = call <vilib>:"Invoke Commands.vi"("Command Params"="Command Params", "Function Name"=w395) -> ("Params"=w391:u8, "Started"=w390:bool)  [unwired: 7 in, 1 out]
        n248 = Array Subset(array="Command Params", length (row)=w391) -> (w392:string[][])  [unwired: 3 in]
        n249 = Select(t="Executing" ("Cmd Status"), s=w390, f="" ("Cmd Status")) -> (s? t:f=→"Cmd Status":string)
      }
      event "Command Selection": Double Click {
        n250 = event-data() -> ("Row"=w405:i32)  [unwired: 1 in]
        n251 = property on="Command Selection" class="MCListbox (strict)"() -> ("ItemNames"=w408:string[][])  [unwired: 2 in, 2 out]
        n252 = local read "Command Params"() -> (w404:string[][])
        n253 = Index Array(array=w408, index (row)=w405, index (col)=0) -> (element=w406:string)
        n254 = call <vilib>:"Invoke Commands.vi"("Command Params"=w404, "Function Name"=w406) -> ("Params"=w403:u8, "Started"=w398:bool)  [unwired: 7 in, 1 out]
        n255 = Array Subset(array=w404, length (row)=w403) -> (w402:string[][])  [unwired: 3 in]
        n256 = Select(t="Executing" ("Cmd Status"), s=w398, f="" ("Cmd Status")) -> (s? t:f=w399:string)
        n257 = local write "Cmd Status"(w399) -> ()
      }
      event "CheckList": Double Click {
        # "Shift clears all"
        # "Update symbols on the listbox"
        n258 = event-data() -> ("PlatMods.Shift"=w410:bool, "Row"=w412:i32)  [unwired: 1 in]
        n259 = case shown="False" w410 {
          tunnel: w412 -> [w416 _]
          tunnel: 1 -> [w415 _]
          frame False {
            n260 = property on="CheckList" class="LstBox (strict)"() -> ("Item Symbols"=w414:i32[])  [unwired: 2 in, 2 out]
            n261 = Replace Array Subset(array=w414, new element=w415, index=w416) -> (w413:i32[])
            n262 = property on="CheckList" class="LstBox (strict)"("Item Symbols"=w413) -> ()  [unwired: 2 in, 2 out]
          }
          frame True {
            w417 = 0 ("Top Row")
            n263 = property on="CheckList" class="LstBox (strict)"() -> ("Number of Rows"=w419:u32)  [unwired: 2 in, 2 out]
            n264 = Initialize Array(0, w419) -> (w418:i32[])
            n265 = property on="CheckList" class="LstBox (strict)"("Top Row"=w417, "Value"=w417, "Item Symbols"=w418) -> ()  [unwired: 2 in, 2 out]
          }
        }
      }
      event "CheckList": Key Down {
        # "Update symbols on the listbox\nLeft and right keys check and uncheck"
        n266 = event-data() -> ("VKey"=w423:T20)  [unwired: 1 in]
        n267 = case shown="\"Left\", \"Right\"" w423 {
          selector: w423 -> [w428 _]
          tunnel: eventvkey."Left" ("VKey") -> [w426 _]
          frame "Left", "Right" {
            n268 = Equal?(x=w426, y=w428) -> (x = y?=w427:bool)
            n269 = Select(t=0, s=w427, f=1) -> (s? t:f=w429:i32)
            n270 = property on="CheckList" class="LstBox (strict)"() -> ("Item Symbols"=w432:i32[])  [unwired: 2 in, 2 out]
            n271 = Replace Array Subset(array=w432, new element=w429, index="CheckList") -> (w431:i32[])
            n272 = property on="CheckList" class="LstBox (strict)"("Item Symbols"=w431) -> ()  [unwired: 2 in, 2 out]
          }
          frame Default {
          }
        }
      }
      event "Motor.Enable": Value Change {
        # "When the test mode otor enable helper is set, update that\ntree row item's value"
        n273 = event-data() -> ("NewVal"=w438:bool)  [unwired: 1 in]
        n274 = Unbundle("Motor") -> ("Value"=w437:dbl)  [unwired: 1 out]
        n275 = Select(t=w437, s=w438, f=0.0) -> (s? t:f=w435:dbl)
        n276 = call <vilib>:"NT Write Number.vi"("Numeric"=w435, "Name"=w434) -> ()  [unwired: 9 in, 1 out]
      }
      event "Test Slider": Value Change {
        # "When the test mode slider helper is set, update that\ntree row item's value"
        n277 = event-data() -> ("NewVal"=w441:dbl)  [unwired: 1 in]
        n278 = call <vilib>:"NT Write Number.vi"("Numeric"=w441, "Name"=w442) -> ()  [unwired: 9 in, 1 out]
      }
      event "On/Off": Value Change {
        # "When the test mode on/off helper value is set, update that\ntree row item's value"
        n279 = event-data() -> ("NewVal"=w446:bool)  [unwired: 1 in]
        n280 = Boolean To (0,1)(Boolean=w446) -> (0, 1=w445:i16)
        n281 = call <vilib>:"NT Write Number.vi"("Numeric"=w445, "Name"=w444) -> ()  [unwired: 9 in, 1 out]
      }
      event "Rev/Fwd": Value Change {
        # "When the test mode helper value for relays is set, update that\ntree row item's value"
        n282 = event-data() -> ("NewVal.Forward"=w454:bool, "NewVal.Reverse"=w453:bool)  [unwired: 1 in]
        n283 = Boolean To (0,1)(Boolean=w454) -> (0, 1=w450:i16)
        n284 = Boolean To (0,1)(Boolean=w453) -> (0, 1=w452:i16)
        n285 = Negate(x=w452) -> (-x=w451:i16)
        n286 = Add(x=w450, y=w451) -> (x+y=w449:i16)
        n287 = call <vilib>:"NT Write Number.vi"("Numeric"=w449, "Name"=w448) -> ()  [unwired: 9 in, 1 out]
      }
      event "Test Ring": Value Change {
        # "When a test mode helper value is selected from the ring,\nset the tree item's variable to the string value"
        n288 = event-data() -> ("NewVal"=w458:u16)  [unwired: 1 in]
        n289 = property on="Test Ring" class="Ring (strict)"() -> ("Strings []"=w459:string[])  [unwired: 2 in, 2 out]
        n290 = Index Array(array=w459, index=w458) -> (element=w457:string)
        n291 = call <vilib>:"NT Write String.vi"("String"=w457, "Name"=w456) -> ()  [unwired: 9 in, 1 out]
      }
      event "Rec Mode": Value Change {
        # "Update globals for recording mode and path to read log from.\nClear when logging and let NetworkTables set path for vision to\nuse."
        n292 = event-data() -> ("NewVal"=w468:enum32{"Stop", "Record", "Playback"})  [unwired: 1 in]
        n293 = global write "WPI_DashboardLogging Global.vi" "Logging Filename"(path "") -> ()
        n294 = global write "WPI_DashboardLogging Global.vi" "Recording"(w468) -> ()
        n295 = case shown="\"Playback\"" w468 {
          tunnel: w467 -> [_ w470 w477]
          tunnel: [_ _ w476] -> w465
          tunnel: [_ _ w475] -> _
          tunnel: w463 -> [_ _ w473]
          tunnel: cluster{i32, i32} {-250, 170} -> [_ _ w472]
          tunnel: w461 -> [_ _ w471]
          frame Default {
          }
          frame "Stop", "Record" {
            # "Place Window too"
            n296 = invoke class="VI" method="FP.Close"(reference=w470) -> (reference out=w469:refnum<vi>)  [unwired: 2 in, 2 out]
            n297 = invoke class="VI" method="Abort VI"(reference=w469) -> ()  [unwired: 2 in, 3 out]
          }
          frame "Playback" {
            n298 = call "Open Playback Panel.vi"("Offset"=w472, "DB VI Ref"=w473, "Playback in"=w477) -> ("Playback out"=w474:refnum<vi>)  [unwired: 8 in]
            n299 = register-events(w474, w471) -> (reference out=w476:refnum<event-registration>, error out=w475:errorcluster)  [unwired: 2 in]
          }
        }
        n300 = call <vilib>:"WPI_DashboardNT Log FieldName Cache.vi"("Operation"=enum16{"Lookup/Add", "Index", "Clear"}."Clear") -> ()  [unwired: 8 in, 3 out]
      }
      event Panel Close {
        w479 = enum32{"Stop", "Record", "Playback"}."Stop" ("Rec Mode")
        # "Playback window has been closed, abort"
        n301 = event-data() -> ()  [unwired: 1 in, 4 out]
        n302 = local write "Rec Mode"(w479) -> ()
        n303 = global write "WPI_DashboardLogging Global.vi" "Recording"(w479) -> ()
      }
      event Panel Close {
        # "Abort playback window and ourself"
        n304 = event-data() -> ()  [unwired: 1 in, 4 out]
        n305 = invoke class="VI" method="FP.Close"(reference=w483) -> (reference out=w482:refnum<vi>)  [unwired: 2 in, 2 out]
        n306 = invoke class="VI" method="Abort VI"(reference=w482) -> (error out=w481:errorcluster)  [unwired: 2 in, 2 out]
        n307 = invoke class="VI" method="Abort VI"(error in=w481) -> ()  [unwired: 2 in, 3 out]
      }
      event User Event {
        n308 = event-data() -> ("IDs"=w490:cluster{"RPC field ID":u16, "Unique ID":u16}, "String"=w489:string)  [unwired: 1 in]
        n309 = Bundle("IDs"=w490, "String"=w489) -> (w488:T10)  [unwired: 1 in]
        n310 = call <vilib>:"Retrieve RPC Response.vi"("RPC Response"=w488) -> ("Output"=w486:string[][])  [unwired: 10 in]
        n311 = Build Array (concatenate)(w484, w486) -> (w485:string[][])
        n312 = local write "Command Params"(w485) -> ()
        n313 = local write "Cmd Status"("" ("Cmd Status")) -> ()
      }
      event "Tree": Double Click {
        n314 = event-data() -> ("PlatMods"=w496:T23, "Tag"=w493:string)  [unwired: 1 in]
        n315 = Unbundle(w496) -> ("Shift"=w495:bool)  [unwired: 4 out]
        n316 = String Subset(string=w493, length (rest)=1 ("length (rest)")) -> (substring=w492:string)  [unwired: 1 in]
        n317 = Not(x=w495) -> (.not. x?=w494:bool)
        n318 = case shown="\"/\"" w492 {
          tunnel: w493 -> [_ w499]
          tunnel: w494 -> [_ w498]
          frame Default {
          }
          frame "/" {
            n319 = call <vilib>:"NT Update Persistence.vi"("Persistence"=w498, "Name"=w499) -> ()  [unwired: 9 in, 1 out]
          }
        }
      }
    }
  }
  n320 = while {
    tunnel: w61 -> [w501]
    i -> [w504]
    stop <- FALSE stop-if-true
    n321 = Wait (ms)(milliseconds to wait=u32 100) -> ()  [unwired: 1 out]
    n322 = case shown="\"Playback\"" "Rec Mode" {
      tunnel: w504 -> [_ _ w519]
      tunnel: [u32 2829099 ("Base Color") u32 11141120 ("Target Color") w508] -> w500
      frame "Stop", Default {
        # "Reset the color, extra updates don't cost much"
      }
      frame "Record" {
      }
      frame "Playback" {
        # "Playback"
        n323 = Quotient & Remainder(x=w519, y=u32 50 ("milliseconds to wait")) -> (x-y*floor(x/y)=w515:u32)  [unwired: 1 out]
        n324 = Divide(x=w515, y=u32 50 ("milliseconds to wait")) -> (x/y=w512:dbl)
        n325 = Multiply(x=6.283185307179586, y=w512) -> (x*y=w517:dbl)
        n326 = Sine(x=w517) -> (sin(x)=w516:dbl)
        n327 = Absolute Value(x=w516) -> (abs(x)=w509:dbl)
        n328 = call "Interpolate RGB Color.vi"("Proportion"=w509, "Target Color"=u32 30976, "Base Color"=u32 2829099) -> ("Result Color"=w508:u32)  [unwired: 8 in]
      }
    }
    n329 = property class="Pane"(reference=w501, "PaneColor"=w500) -> ()  [unwired: 1 in, 2 out]
  }
  n330 = property on="On/Off" class="Bool (strict)"("Visible"=w34) -> ()  [unwired: 2 in, 2 out]
  n331 = property on="Motor" class="Clust (strict)"("Visible"=w34) -> ()  [unwired: 2 in, 2 out]
  n332 = property on="Progress" class="Clust (strict)"("Visible"=w34) -> ()  [unwired: 2 in, 2 out]
  n333 = property on="Test Ring" class="Ring (strict)"("Visible"=w34) -> ()  [unwired: 2 in, 2 out]
  n334 = property on="Rev/Fwd" class="Clust (strict)"("Visible"=w34) -> ()  [unwired: 2 in, 2 out]
  n335 = while {
    tunnel: u16 1741 ("timeout ms (25000)") -> [w521]
    stop <- FALSE stop-if-true
    n336 = TCP Create Listener(10:w521) -> (0:w520:errorcluster, 3:w522:refnum<k5>)  [unwired: 4 in, 1 out]
    n337 = case shown="No Error" w520 {
      selector: w520 -> [w524 _]
      tunnel: w522 -> [w525 _]
      frame No Error {
        n338 = while {
          tunnel: w525 -> [w528]
          tunnel: w524 -> [w527]
          stop <- FALSE stop-if-true
          n339 = TCP Wait On Listener(8:w527, 11:w528) -> (0:w529:errorcluster, 4:w530:refnum<k5>)  [unwired: 2 in, 3 out]
          n340 = local write "TCP"(w530) -> ()
          n341 = case shown="No Error" w529 {
            frame No Error {
            }
            frame Error {
              n342 = Wait (ms)(milliseconds to wait=u32 1000) -> ()  [unwired: 1 out]
            }
          }
        }
      }
      frame Error {
        n343 = Wait (ms)(milliseconds to wait=u32 1000) -> ()  [unwired: 1 out]
      }
    }
  }
  n344 = local write "Command Selection"(u16 0 ("milliseconds to wait")) -> ()
  n345 = local write "Command Params"(string[][] [] ("Command Params")) -> ()
  n346 = global write "WPI_DashboardLogging Global.vi" "Recording"(w55) -> ()
  n347 = local write "Rec Mode"(w55) -> ()
  n348 = call <vilib>:"NT Write String.vi"("String"="Select Auto", "Name"="Auto Selector") -> ()  [unwired: 9 in, 1 out]
